vi "Write to Log.vi"(8 "error in (no error)":errorcluster, 10 "Text to Write":string, 11 "String Indicator Logger in":refnum<class "String Indicator Logger.lvclass">) -> (0 "error out":errorcluster, 3 "String Indicator Logger out":refnum<class "String Indicator Logger.lvclass">)   [LabVIEW 2020, in "String Indicator Logger.lvclass"]
uses:
  String Indicator Logger.lvclass
  String Indicator Logger.lvclass/String Indicator Logger.ctl
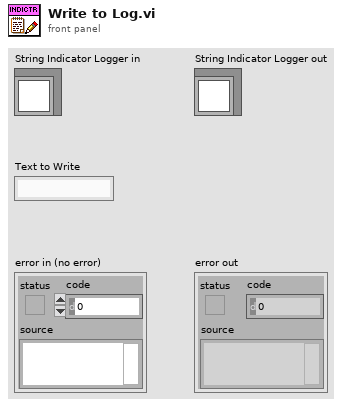
[diagram p1: front panel]
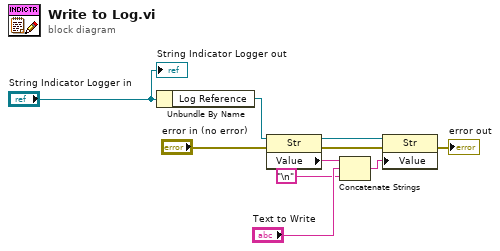
[diagram p0: block diagram]
diagram:
  n1 = Unbundle By Name("String Indicator Logger in") -> ("Log Reference"=w9:refnum<vi>)
  n2 = property class="Str"(reference=w9, error in="error in (no error)") -> (reference out=w7:refnum<vi>, error out=w4:errorcluster, "Value"=w8:string)
  n3 = Concatenate Strings(w8, "Text to Write", "\n") -> (w6:string)
  n4 = property class="Str"(reference=w7, error in=w4, "Value"=w6) -> (error out=→"error out":errorcluster)  [unwired: 1 out]
  "String Indicator Logger out" <- "String Indicator Logger in"
